vi "ToggleMode.vi"(8 "error in (no error)":errorcluster, 10 "Mode":T1, 11 "Drive in":refnum<class "Drive.lvclass">) -> (0 "error out":errorcluster, 3 "Drive out":refnum<class "Drive.lvclass">)   [LabVIEW 2019, in "DriveOld.lvlib" / "Drive.lvclass"]
doc: "Configures the talons based on weather your running closed loop velocity mode or motion magic"
uses:
  Drive.lvclass
  Pod Drive/Controls/Mode.ctl
  Pod Drive/Pod Drive.lvclass
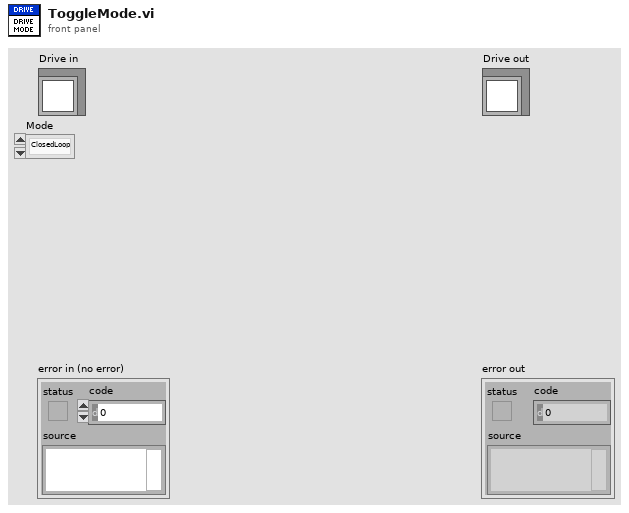
[diagram p1: front panel]
types:
  T1 = typedef "DriveOld.lvlib/Pod Drive.lvclass/Mode.ctl" = enum16{"ClosedLoop", "MotionMagic"}
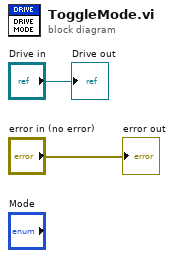
[diagram p0: block diagram]
diagram:
  "error out" <- "error in (no error)"
  "Drive out" <- "Drive in"
